vi "CRM Admin panel.vi"() -> ()   [LabVIEW 2016]
uses:
  Typedef/CRM Admin - States.ctl
  Typedef/CRM Admin - Tab options.ctl
  Typedef/Device data.ctl
  Typedef/MAC & Labels.ctl
  <vilib>/httpClient/POSTBuffer.vi
  <vilib>/httpClient/LabVIEWHTTPClient.lvlib
panel:
  in  "Exit":bool
  in  "Tab Control":T1(tab)
  in  "Refresh":bool
  out "Temp Plot":cluster{dbl[], dbl[]}[](graph)
  out "Hum Plot":cluster{dbl[], dbl[]}[](graph)
  in  "Update labels":bool
  in  "Device List":i32(listbox)
  in  "Set parameters":bool
  in  "Alert setting":T2 {"Temperature High" format="%#.2g°C"; "Humidity High" format="%#.2g%"; "Low battery" min=0.0 max=4.2 step=0.05 format="%#.2gV"; "Temperature Low" format="%#.2g°C"; "Humidity Low" format="%#.2g%"}
  # "Alert Threshold"
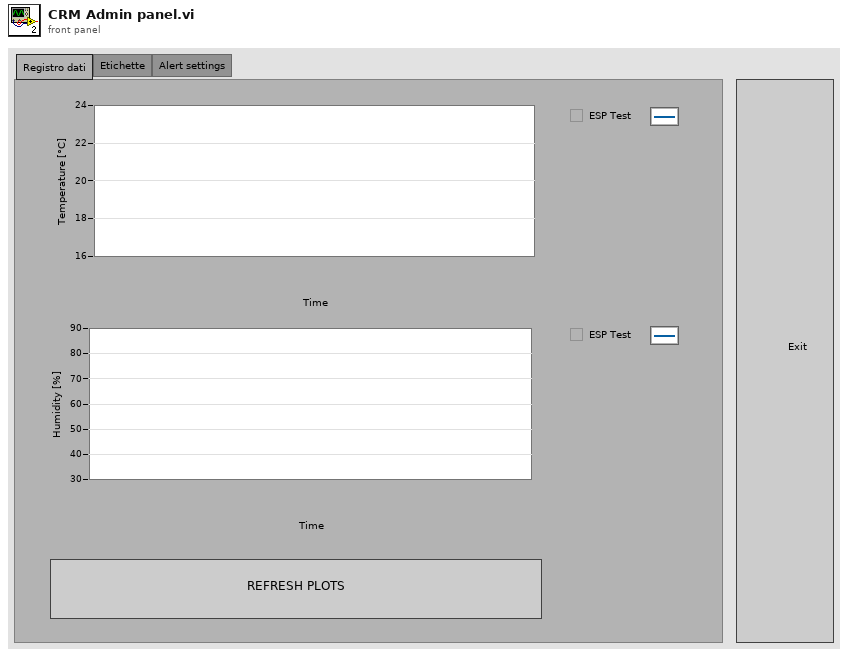
[diagram p1: front panel]
types:
  T1 = enum32{"Registro dati", "Etichette", "Alert settings"}
  T2 = cluster{"Mail recipients":string[], "Enable":bool, "Low battery":dbl, "Temperature Low":dbl, "Humidity Low":dbl, "Humidity High":dbl, "Temperature High":dbl}
  T3 = typedef "CRM Admin - States.ctl" = enum16{"Read LastData", "Get Labels", "Set Labels", "Set Alert parameters", "Exit"}
  T4 = typedef "CRM Admin - Tab options.ctl" = enum32{"Registro dati", "Etichette", "Alert settings"}
  T5 = typedef "LabVIEWHTTPClient.lvlib/ClientHandle.ctl" = refnum<k1>
  T6 = typedef "Device data.ctl" = cluster{"MAC Address":string, "Label":string, "Data":dbl[][]}
  T7 = typedef "MAC & Labels.ctl" = cluster{"MAC list":string[], "Label list":string[]}
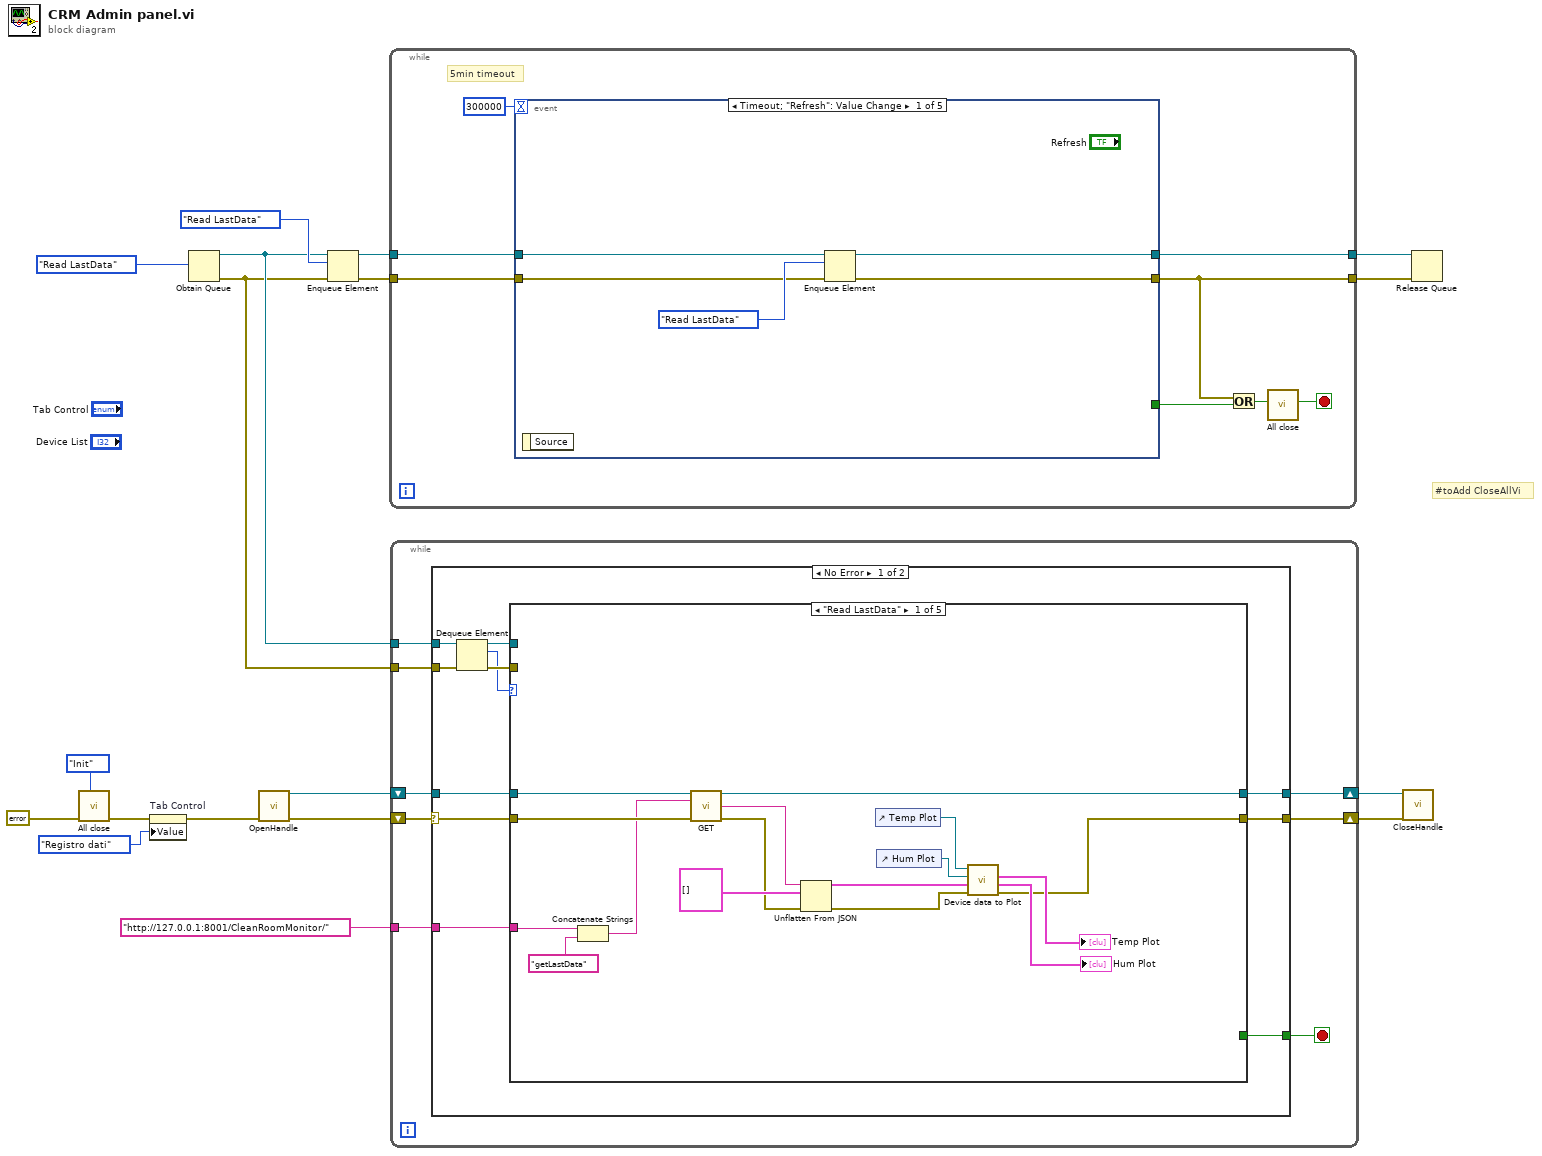
[diagram p0: block diagram]
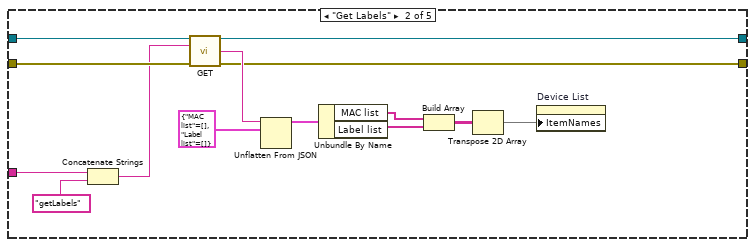
[diagram p2: hidden frame]
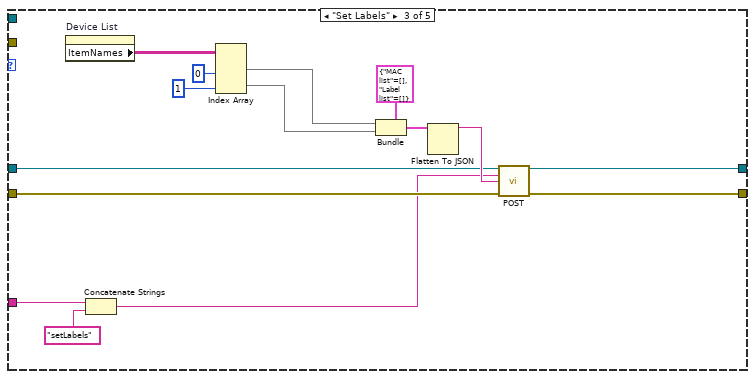
[diagram p3: hidden frame]
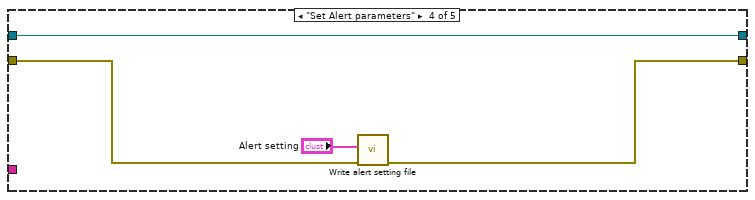
[diagram p4: hidden frame]
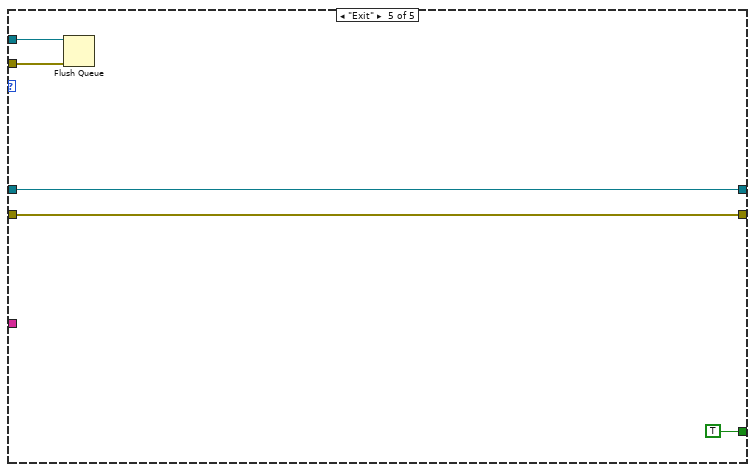
[diagram p5: hidden frame]
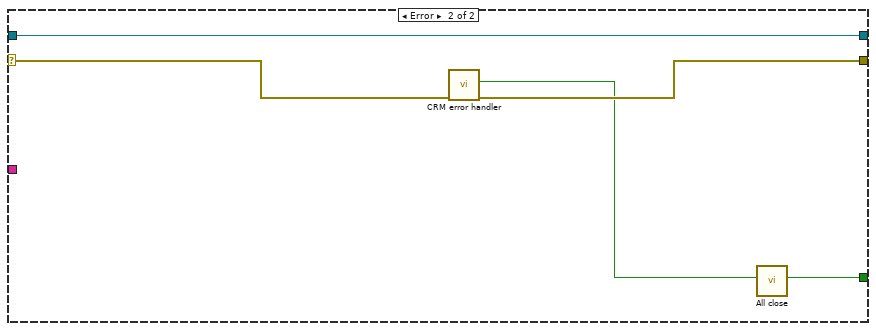
[diagram p6: hidden frame]
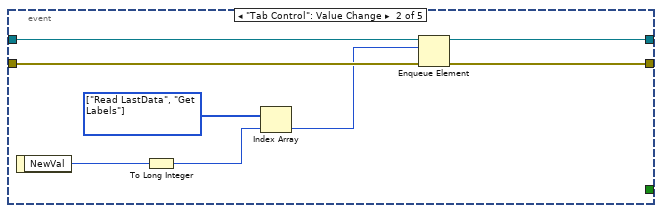
[diagram p7: hidden frame]
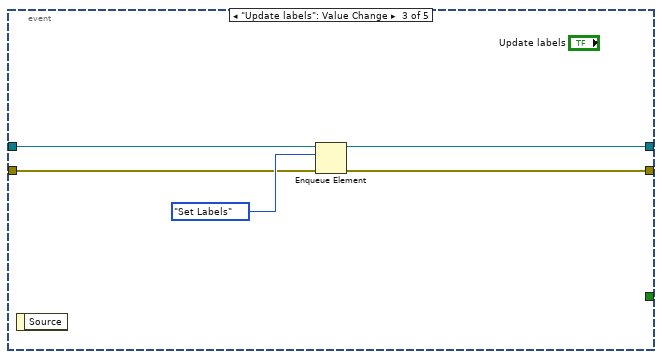
[diagram p8: hidden frame]
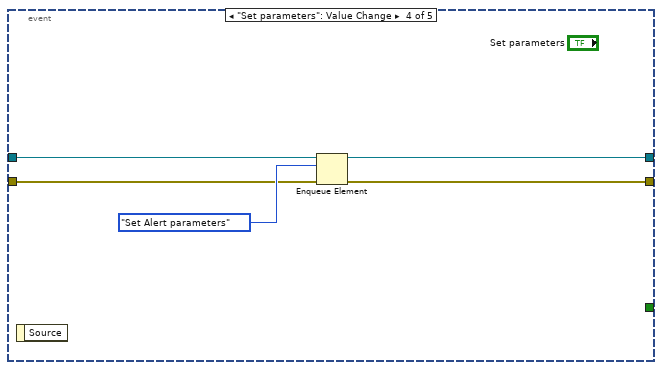
[diagram p9: hidden frame]
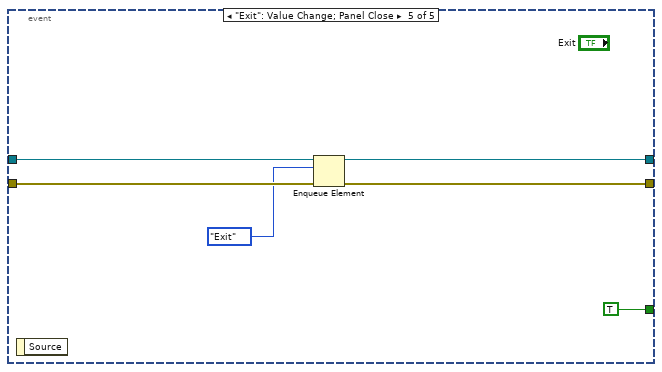
[diagram p10: hidden frame]
diagram:
  # "#toAdd CloseAllVi"
  n1 = call "All close.vi"("Operation (Check)"=enum16{"Init", "Check"}."Init", "Error In"=errorcluster {"status"=FALSE, "code"=0, "source"=""} ("error in (no error)")) -> ("Error Out"=w1:errorcluster)  [unwired: 8 in, 1 out]
  n2 = property on="Tab Control" class="TabCtl (strict)"(error in=w1, "Value"=CRM_Admin_-_Tab_options."Registro dati" ("Tab Control")) -> (error out=w16:errorcluster)  [unwired: 1 in, 1 out]
  n3 = Obtain Queue(element data type=CRM_Admin_-_States."Read LastData") -> (queue out=w5:refnum<queue>, error out=w4:errorcluster)  [unwired: 4 in, 1 out]
  n4 = call <vilib>:"OpenHandle.vi"("error in (no error)"=w16) -> ("client handle out"=w15:T5, "error out"=w14:errorcluster)  [unwired: 13 in]
  n5 = Enqueue Element(queue=w5, element=CRM_Admin_-_States."Read LastData", error in (no error)=w4) -> (queue out=w7:refnum<queue>, error out=w6:errorcluster)  [unwired: 1 in, 1 out]
  n6 = while {
    tunnel: w7 -> [w26]
    tunnel: w6 -> [w25]
    tunnel: [w24] -> w18
    tunnel: [w23] -> w17
    stop <- w19 stop-if-true
    # "5min timeout"
    n7 = event shown="[0] Timeout;  \"Refresh\": Value Change" {
      selector: _ -> [_ _ _ _ _]
      dyn-events: _ -> [_ _ _ _ _]
      timeout: 300000 -> [_ _ _ _ _]
      tunnel: w26 -> [w30 w39 w43 w48 w54]
      tunnel: w25 -> [w29 w38 w42 w47 w52]
      tunnel: [w28 w36 w40 w45 w53] -> w24
      tunnel: [w27 w37 w41 w46 w51] -> w23
      tunnel: [_ _ _ _ TRUE] -> w22
      event Timeout; "Refresh": Value Change {
        n8 = event-data() -> ()  [unwired: 1 in, 1 out]
        n9 = Enqueue Element(queue=w30, element=CRM_Admin_-_States."Read LastData", error in (no error)=w29) -> (queue out=w28:refnum<queue>, error out=w27:errorcluster)  [unwired: 1 in, 1 out]
      }
      event "Tab Control": Value Change {
        w35 = T3[] [enum."Read LastData", enum."Get Labels"] items=["Read LastData", "Get Labels", "Set Labels", "Set Alert parameters", "Exit"]
        n10 = event-data() -> ("NewVal"=w34:T1)  [unwired: 1 in]
        n11 = To Long Integer(number=w34) -> (32bit integer=w33:i32)
        n12 = Index Array(array=w35, index=w33) -> (element=w32:T3)
        n13 = Enqueue Element(queue=w39, element=w32, error in (no error)=w38) -> (queue out=w36:refnum<queue>, error out=w37:errorcluster)  [unwired: 1 in, 1 out]
      }
      event "Update labels": Value Change {
        n14 = event-data() -> ()  [unwired: 1 in, 1 out]
        n15 = Enqueue Element(queue=w43, element=CRM_Admin_-_States."Set Labels", error in (no error)=w42) -> (queue out=w40:refnum<queue>, error out=w41:errorcluster)  [unwired: 1 in, 1 out]
      }
      event "Set parameters": Value Change {
        n16 = event-data() -> ()  [unwired: 1 in, 1 out]
        n17 = Enqueue Element(queue=w48, element=CRM_Admin_-_States."Set Alert parameters", error in (no error)=w47) -> (queue out=w45:refnum<queue>, error out=w46:errorcluster)  [unwired: 1 in, 1 out]
      }
      event "Exit": Value Change; Panel Close {
        n18 = event-data() -> ()  [unwired: 1 in, 1 out]
        n19 = Enqueue Element(queue=w54, element=CRM_Admin_-_States."Exit", error in (no error)=w52) -> (queue out=w53:refnum<queue>, error out=w51:errorcluster)  [unwired: 1 in, 1 out]
      }
    }
    n20 = Or(x=w23, y=w22) -> (x .or. y?=w20:bool)
    n21 = call "All close.vi"("Close? (F)"=w20) -> ("Close"=w19:bool)  [unwired: 9 in, 1 out]
  }
  n22 = while {
    shift-right: [w61] -> w12
    shift-left: w15 -> [w62]
    shift-right: [w60] -> w11
    shift-left: w14 -> [w63]
    tunnel: w5 -> [w56]
    tunnel: w4 -> [w57]
    tunnel: "http://127.0.0.1:8001/CleanRoomMonitor/" ("url") -> [w58]
    stop <- w59 stop-if-true
    n23 = case shown="No Error" w63 {
      selector: w63 -> [w73 w132]
      tunnel: w56 -> [w68 _]
      tunnel: w57 -> [w67 _]
      tunnel: w62 -> [w74 w133]
      tunnel: [w72 w133] -> w61
      tunnel: [w71 w131] -> w60
      tunnel: [w70 w129] -> w59
      tunnel: w58 -> [w69 _]
      frame No Error {
        n24 = Dequeue Element(queue=w68, error in (no error)=w67) -> (queue out=w65:refnum<queue>, element=w64:T3, error out=w66:errorcluster)  [unwired: 1 in, 1 out]
        n25 = case shown="\"Read LastData\"" w64 {
          tunnel: w65 -> [_ _ _ _ w128]
          tunnel: w66 -> [_ _ _ _ w127]
          tunnel: w74 -> [w81 w101 w114 w123 w126]
          tunnel: w73 -> [w80 w100 w113 w122 w125]
          tunnel: [w79 w98 w116 w123 w126] -> w72
          tunnel: [w76 w99 w115 w121 w125] -> w71
          tunnel: [_ _ _ _ TRUE] -> w70
          tunnel: w69 -> [w89 w96 w111 _ _]
          frame "Read LastData" {
            n26 = Concatenate Strings(w89, "getLastData" ("url")) -> (w78:string)
            n27 = call <vilib>:"GET.vi"("client handle"=w81, "url"=w78, "error in (no error)"=w80) -> ("client handle out"=w79:T5, "body"=w82:string, "error out"=w77:errorcluster)  [unwired: 9 in, 1 out]
            n28 = Unflatten From JSON(JSON string=w82, type and defaults=T6[] [], error in (no error)=w77) -> (value=w84:T6[], error out=w75:errorcluster)  [unwired: 4 in]
            n29 = control-ref of="Temp Plot"() -> (w85:refnum<vi>)
            n30 = control-ref of="Hum Plot"() -> (w86:refnum<vi>)
            n31 = call "Device data to Plot.vi"("Error In"=w75, "Device Data array"=w84, "Hum Plot Reference"=w86, "Temp Plot Reference"=w85) -> ("Error Out"=w76:errorcluster, "Hum Plot"=→"Hum Plot":cluster{"Array":dbl[], "Array":dbl[]}[], "Temp Plot"=→"Temp Plot":cluster{"Array":dbl[], "Array":dbl[]}[])  [unwired: 5 in]
          }
          frame "Get Labels" {
            n32 = Concatenate Strings(w96, "getLabels" ("url")) -> (w95:string)
            n33 = call <vilib>:"GET.vi"("client handle"=w101, "url"=w95, "error in (no error)"=w100) -> ("client handle out"=w98:T5, "body"=w102:string, "error out"=w99:errorcluster)  [unwired: 9 in, 1 out]
            n34 = Unflatten From JSON(JSON string=w102, type and defaults=T7 {"MAC list"=[], "Label list"=[]} ("MAC-label")) -> (value=w104:T7)  [unwired: 5 in, 1 out]
            n35 = Unbundle By Name(w104) -> ("MAC list"=w94:string[], "Label list"=w93:string[])
            n36 = Build Array(w94, w93) -> (w92:string[][])
            n37 = Transpose 2D Array(2D array=w92) -> (transposed array=w91:string[][])
            n38 = property on="Device List" class="MCListbox (strict)"("ItemNames"=w91) -> ()  [unwired: 2 in, 2 out]
          }
          frame "Set Labels" {
            n39 = property on="Device List" class="MCListbox (strict)"() -> ("ItemNames"=w109:string[][])  [unwired: 2 in, 2 out]
            n40 = Concatenate Strings(w111, "setLabels" ("url")) -> (w110:string)
            n41 = Index Array(array=w109, index (col) #1=0 ("disabled index (col)"), index (col) #2=1 ("index (col)")) -> (element #1=w106:string[], element #2=w105:string[])  [unwired: 2 in]
            n42 = Bundle(cluster=T7 {"MAC list"=[], "Label list"=[]} ("MAC-label"), "MAC list"=w106, "Label list"=w105) -> (w117:T7)
            n43 = Flatten To JSON(anything=w117) -> (JSON string=w119:string)  [unwired: 2 in, 1 out]
            n44 = call-poly <vilib>:"POST.vi"("client handle"=w114, "url"=w110, "buffer"=w119, "error in (no error)"=w113) -> ("client handle out"=w116:T5, "error out"=w115:errorcluster)  [unwired: 8 in, 2 out]
          }
          frame "Set Alert parameters" {
            n45 = call "Write alert setting file.vi"("Error In"=w122, "Alert setting"="Alert setting") -> ("Error Out"=w121:errorcluster)  [unwired: 9 in]
          }
          frame "Exit" {
            n46 = Flush Queue(queue=w128, error in (no error)=w127) -> ()  [unwired: 3 out]
          }
        }
      }
      frame Error {
        n47 = call "CRM error handler.vi"("Error In"=w132) -> ("Error Out"=w131:errorcluster, "Exit?"=w130:bool)  [unwired: 9 in]
        n48 = call "All close.vi"("Close? (F)"=w130) -> ("Close"=w129:bool)  [unwired: 9 in, 1 out]
      }
    }
  }
  n49 = call <vilib>:"CloseHandle.vi"("client handle"=w12, "error in (no error)"=w11) -> ()  [unwired: 13 in, 1 out]
  n50 = Release Queue(queue=w18, error in (no error)=w17) -> ()  [unwired: 1 in, 3 out]
